vi "BRig_RT__Case_Exp__State_initTrial__LC_ENL__v3.vi"(6 "input_arrTrig":bool[](array[boolean]), 8 "input_dataTrial":u16[][](array[numeric]), 9 "input_dataExp":u16[](array[numeric]), 10 "input_dataLC":u16[](array[numeric]), 11 "input_dataCurrent":u16[](array[numeric])) -> (0 "output_dataTrial":u16[][](array[numeric]), 3 "output_dataCurrent":u16[](array[numeric]), 4 "output_arrTrig":bool[](array[boolean]))   [LabVIEW 2014]
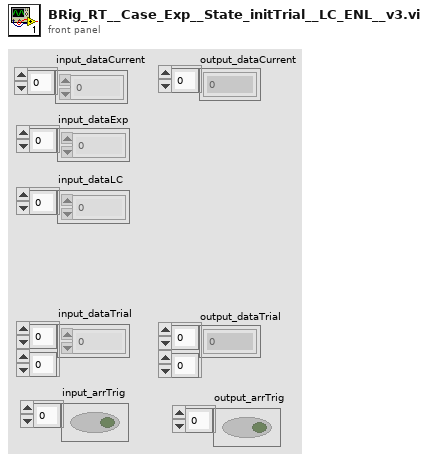
[diagram p1: front panel]
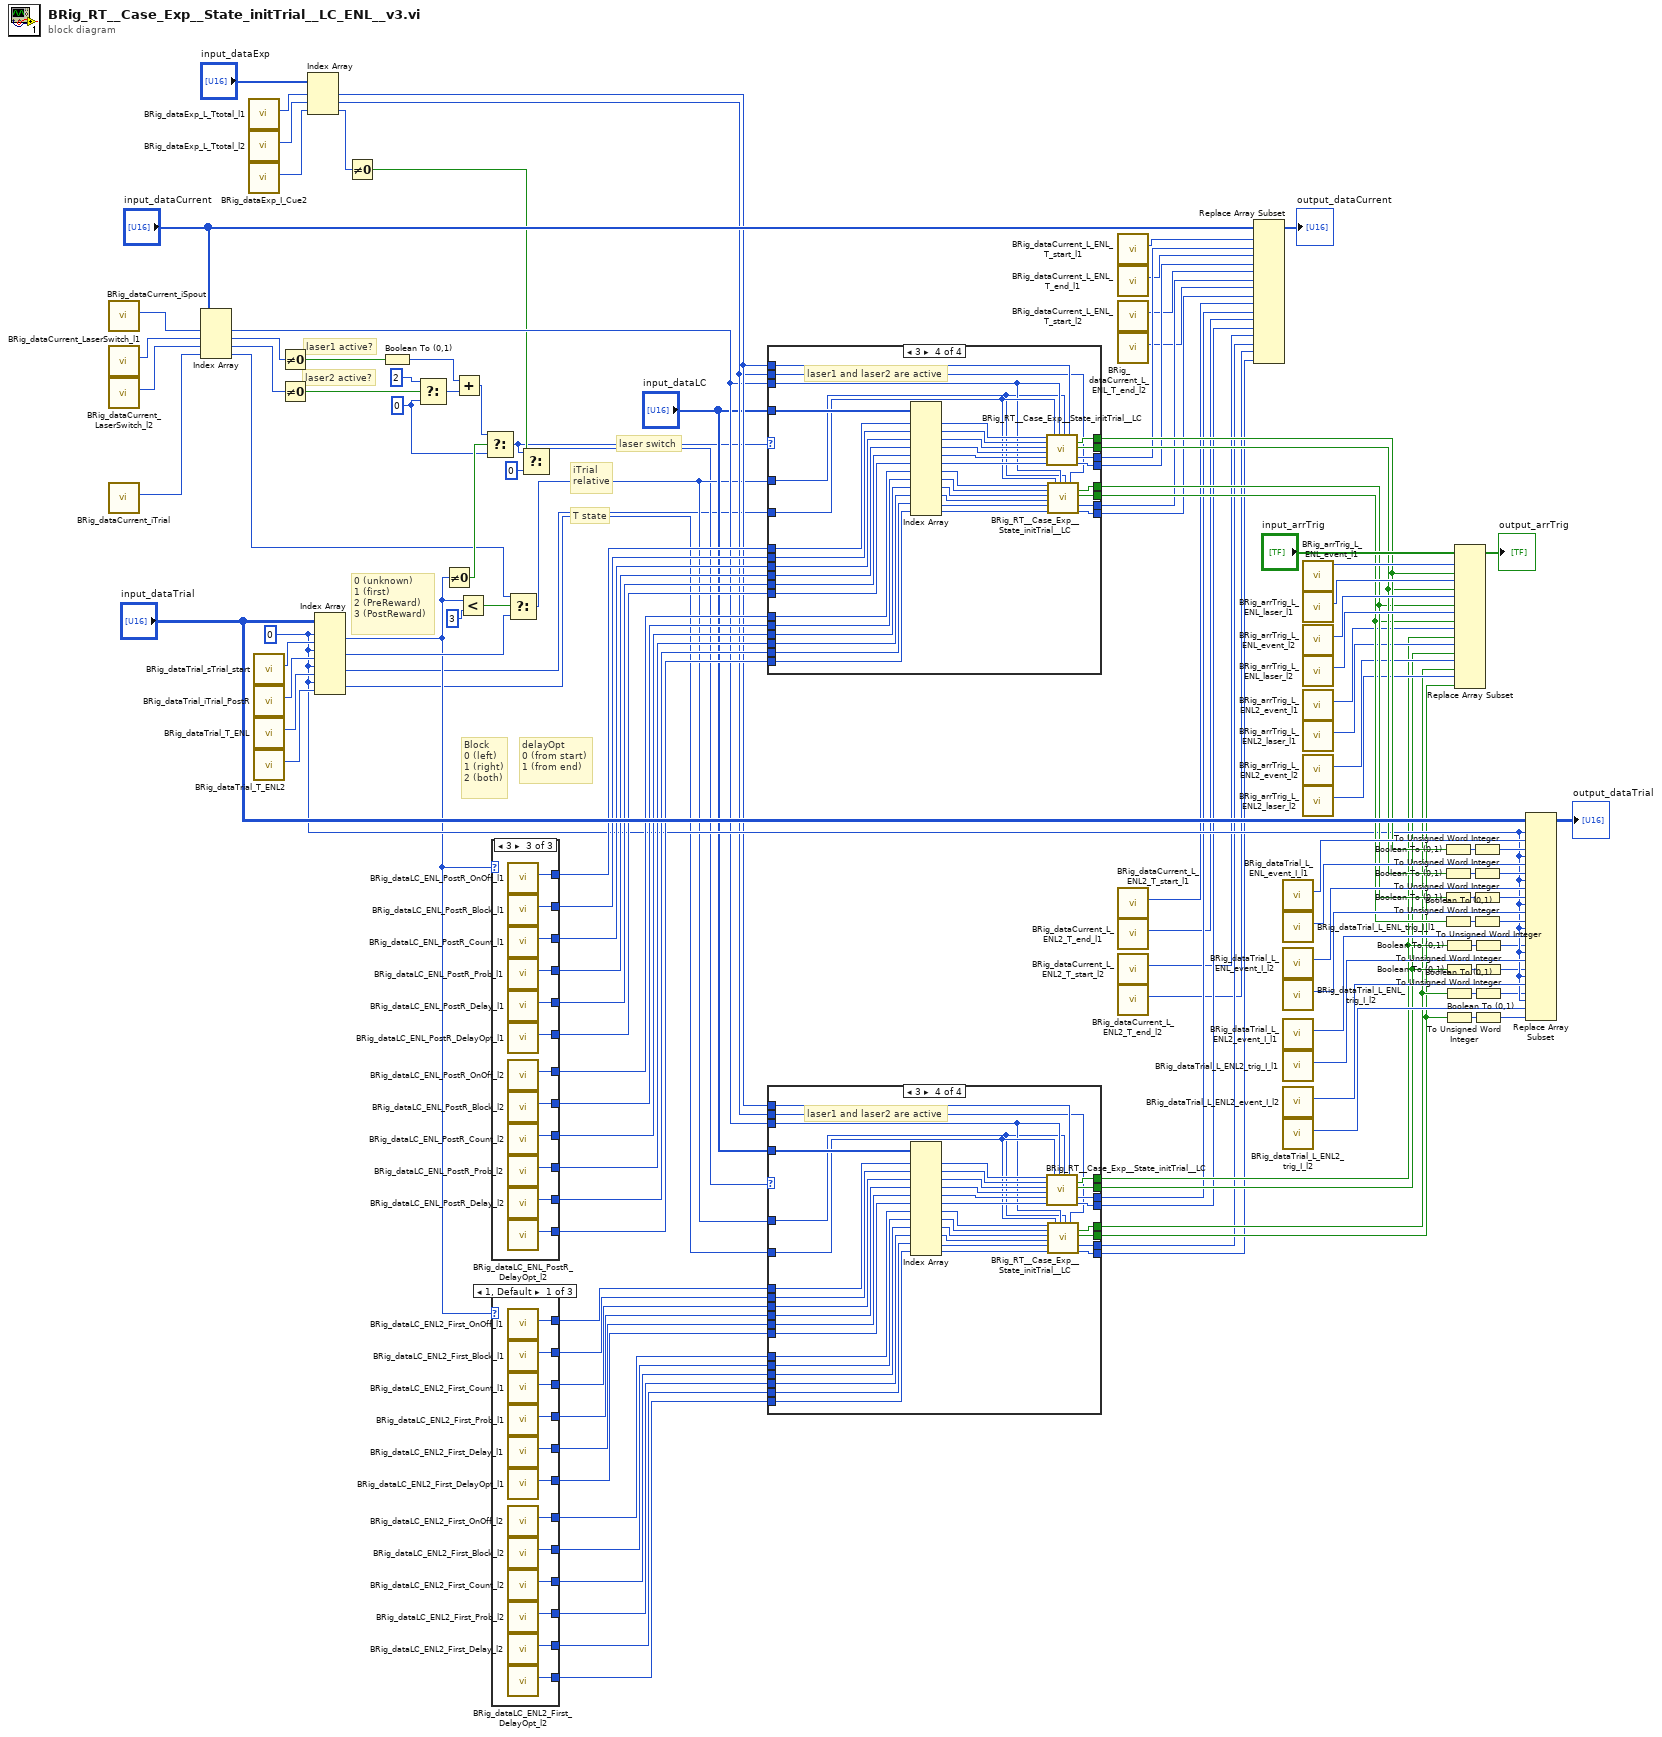
[diagram p0: block diagram]
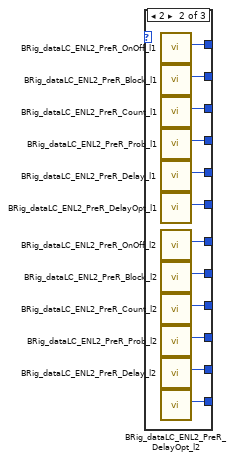
[diagram p2: hidden frame]
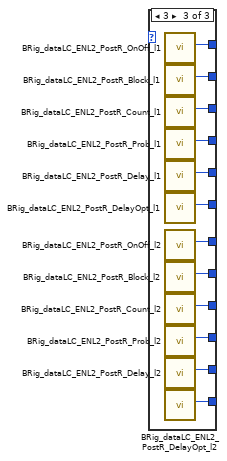
[diagram p3: hidden frame]
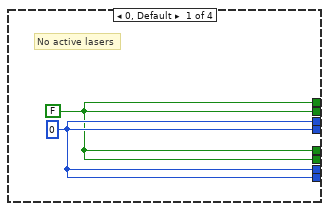
[diagram p4: hidden frame]
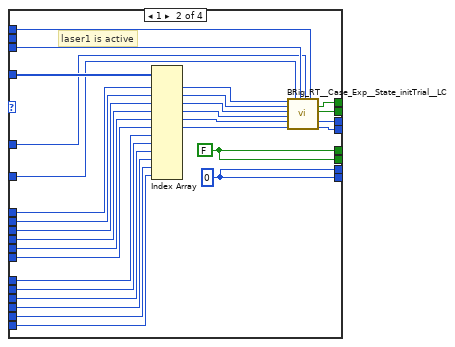
[diagram p5: hidden frame]
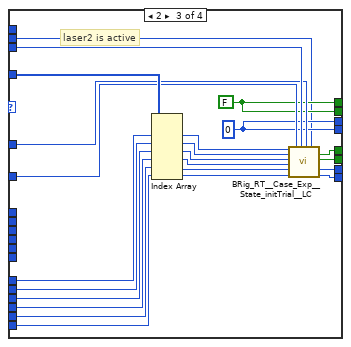
[diagram p6: hidden frame]
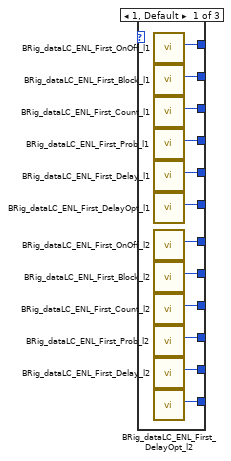
[diagram p7: hidden frame]
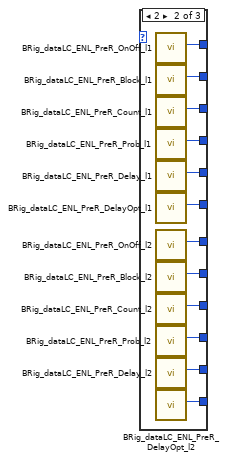
[diagram p8: hidden frame]
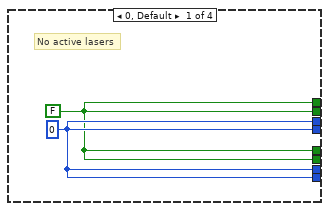
[diagram p9: hidden frame]
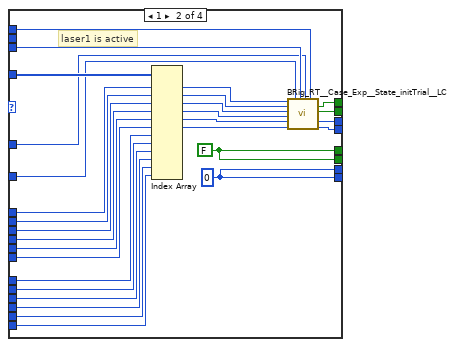
[diagram p10: hidden frame]
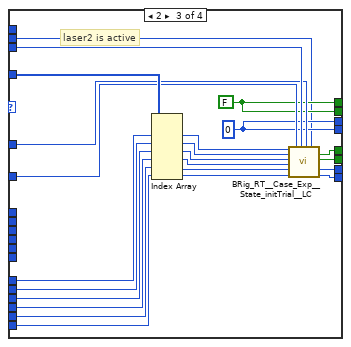
[diagram p11: hidden frame]
diagram:
  w44 = 0
  w115 = i16 0 ("f")
  # "iTrial\nrelative"
  # "laser switch"
  # "T state"
  # "delayOpt\n0 (from start)\n1 (from end)"
  # "Block\n0 (left)\n1 (right)\n2 (both)"
  # "0 (unknown)\n1 (first)\n2 (PreReward)\n3 (PostReward)"
  # "laser2 active?"
  # "laser1 active?"
  n1 = call "BRig_dataCurrent_iSpout.vi"() -> ("output_iSpout"=w113:i32)  [unwired: 11 in]
  n2 = call "BRig_dataCurrent_LaserSwitch_l1.vi"() -> ("output_LaserSwitch_l1"=w126:i32)  [unwired: 11 in]
  n3 = call "BRig_dataCurrent_LaserSwitch_l2.vi"() -> ("output_LaserSwitch_l2"=w125:i32)  [unwired: 11 in]
  n4 = call "BRig_dataCurrent_iTrial.vi"() -> ("output_iTrial"=w58:i32)  [unwired: 11 in]
  n5 = Index Array(array="input_dataCurrent", index #1=w113, index #2=w126, index #3=w125, index #4=w58) -> (element #1=w36:u16, element #2=w124:u16, element #3=w123:u16, element #4=w57:u16)
  n6 = call "BRig_dataExp_L_Ttotal_l1.vi"() -> ("output_L_Ttotal_l1"=w64:i32)  [unwired: 11 in]
  n7 = call "BRig_dataExp_L_Ttotal_l2.vi"() -> ("output_L_Ttotal_l2"=w65:i32)  [unwired: 11 in]
  n8 = call "BRig_dataExp_I_Cue2.vi"() -> ("output_I_Cue2"=w8:i32)  [unwired: 11 in]
  n9 = call "BRig_dataTrial_sTrial_start.vi"() -> ("output_sTrial_start"=w122:i32)  [unwired: 11 in]
  n10 = call "BRig_dataTrial_iTrial_PostR.vi"() -> ("output_iTrial_PostR"=w61:i32)  [unwired: 11 in]
  n11 = call "BRig_dataTrial_T_ENL.vi"() -> ("output_T_ENL"=w62:i32)  [unwired: 11 in]
  n12 = call "BRig_dataTrial_T_ENL2.vi"() -> ("output_T_ENL2"=w56:i32)  [unwired: 11 in]
  n13 = Not Equal To 0?(x=w124) -> (x != 0?=w121:bool)
  n14 = Not Equal To 0?(x=w123) -> (x != 0?=w120:bool)
  n15 = Index Array(array="input_dataExp", index #1=w64, index #2=w65, index #3=w8) -> (element #1=w38:u16, element #2=w37:u16, element #3=w7:u16)
  n16 = Index Array(array="input_dataTrial", index (row) #1=w44, index (col) #1=w122, index (row) #2=w44, index (col) #2=w61, index (row) #3=w44, index (col) #3=w62, index (row) #4=w44, index (col) #4=w56) -> (element #1=w33:u16, element #2=w59:u16, element #3=w2:u16, element #4=w1:u16)
  n17 = Not Equal To 0?(x=w7) -> (x != 0?=w6:bool)
  n18 = Boolean To (0,1)(Boolean=w121) -> (0, 1=w117:i16)
  n19 = Select(t=i16 2, s=w120, f=w115) -> (s? t:f=w118:i16)
  n20 = Not Equal To 0?(x=w33) -> (x != 0?=w116:bool)
  n21 = Add(x=w117, y=w118) -> (x+y=w114:i16)
  n22 = Less?(x=w33, y=u16 3) -> (x < y?=w60:bool)
  n23 = Select(t=w114, s=w116, f=w115) -> (s? t:f=w4:i16)
  n24 = case shown="3" w33 {
    tunnel: [w138 w150 w162] -> w77
    tunnel: [w137 w149 w151] -> w76
    tunnel: [w136 w148 w152] -> w75
    tunnel: [w135 w147 w153] -> w74
    tunnel: [w134 w146 w154] -> w73
    tunnel: [w133 w145 w155] -> w72
    tunnel: [w132 w144 w161] -> w71
    tunnel: [w131 w143 w160] -> w70
    tunnel: [w130 w142 w159] -> w69
    tunnel: [w129 w141 w158] -> w68
    tunnel: [w128 w140 w157] -> w67
    tunnel: [w127 w139 w156] -> w66
    frame 1, Default {
      n25 = call "BRig_dataLC_ENL_First_OnOff_l1.vi"() -> ("output_ENL_First_OnOff"=w138:i32)  [unwired: 11 in]
      n26 = call "BRig_dataLC_ENL_First_Block_l1.vi"() -> ("output_ENL_First_Block"=w137:i32)  [unwired: 11 in]
      n27 = call "BRig_dataLC_ENL_First_Count_l1.vi"() -> ("output_ENL_First_Count"=w136:i32)  [unwired: 11 in]
      n28 = call "BRig_dataLC_ENL_First_Prob_l1.vi"() -> ("output_ENL_First_Prob"=w135:i32)  [unwired: 11 in]
      n29 = call "BRig_dataLC_ENL_First_Delay_l1.vi"() -> ("output_ENL_First_Delay"=w134:i32)  [unwired: 11 in]
      n30 = call "BRig_dataLC_ENL_First_DelayOpt_l1.vi"() -> ("output_ENL_First_DelayOpt"=w133:i32)  [unwired: 11 in]
      n31 = call "BRig_dataLC_ENL_First_OnOff_l2.vi"() -> ("output_ENL_First_OnOff_l2"=w132:i32)  [unwired: 11 in]
      n32 = call "BRig_dataLC_ENL_First_Block_l2.vi"() -> ("output_ENL_First_Block_l2"=w131:i32)  [unwired: 11 in]
      n33 = call "BRig_dataLC_ENL_First_Count_l2.vi"() -> ("output_ENL_First_Count_l2"=w130:i32)  [unwired: 11 in]
      n34 = call "BRig_dataLC_ENL_First_Prob_l2.vi"() -> ("output_ENL_First_Prob_l2"=w129:i32)  [unwired: 11 in]
      n35 = call "BRig_dataLC_ENL_First_Delay_l2.vi"() -> ("output_ENL_First_Delay_l2"=w128:i32)  [unwired: 11 in]
      n36 = call "BRig_dataLC_ENL_First_DelayOpt_l2.vi"() -> ("output_ENL_First_DelayOpt_l2"=w127:i32)  [unwired: 11 in]
    }
    frame 2 {
      n37 = call "BRig_dataLC_ENL_PreR_OnOff_l1.vi"() -> ("output_ENL_PreR_OnOff"=w150:i32)  [unwired: 11 in]
      n38 = call "BRig_dataLC_ENL_PreR_Block_l1.vi"() -> ("output_ENL_PreR_Block"=w149:i32)  [unwired: 11 in]
      n39 = call "BRig_dataLC_ENL_PreR_Count_l1.vi"() -> ("output_ENL_PreR_Count"=w148:i32)  [unwired: 11 in]
      n40 = call "BRig_dataLC_ENL_PreR_Prob_l1.vi"() -> ("output_ENL_PreR_Prob"=w147:i32)  [unwired: 11 in]
      n41 = call "BRig_dataLC_ENL_PreR_Delay_l1.vi"() -> ("output_ENL_PreR_Delay"=w146:i32)  [unwired: 11 in]
      n42 = call "BRig_dataLC_ENL_PreR_DelayOpt_l1.vi"() -> ("output_ENL_PreR_DelayOpt"=w145:i32)  [unwired: 11 in]
      n43 = call "BRig_dataLC_ENL_PreR_OnOff_l2.vi"() -> ("output_ENL_PreR_OnOff_l2"=w144:i32)  [unwired: 11 in]
      n44 = call "BRig_dataLC_ENL_PreR_Block_l2.vi"() -> ("output_ENL_PreR_Block_l2"=w143:i32)  [unwired: 11 in]
      n45 = call "BRig_dataLC_ENL_PreR_Count_l2.vi"() -> ("output_ENL_PreR_Count_l2"=w142:i32)  [unwired: 11 in]
      n46 = call "BRig_dataLC_ENL_PreR_Prob_l2.vi"() -> ("output_ENL_PreR_Prob_l2"=w141:i32)  [unwired: 11 in]
      n47 = call "BRig_dataLC_ENL_PreR_Delay_l2.vi"() -> ("output_ENL_PreR_Delay_l2"=w140:i32)  [unwired: 11 in]
      n48 = call "BRig_dataLC_ENL_PreR_DelayOpt_l2.vi"() -> ("output_ENL_PreR_DelayOpt_l2"=w139:i32)  [unwired: 11 in]
    }
    frame 3 {
      n49 = call "BRig_dataLC_ENL_PostR_OnOff_l1.vi"() -> ("output_ENL_PostR_OnOff"=w162:i32)  [unwired: 11 in]
      n50 = call "BRig_dataLC_ENL_PostR_Block_l1.vi"() -> ("output_ENL_PostR_Block"=w151:i32)  [unwired: 11 in]
      n51 = call "BRig_dataLC_ENL_PostR_Count_l1.vi"() -> ("output_ENL_PostR_Count"=w152:i32)  [unwired: 11 in]
      n52 = call "BRig_dataLC_ENL_PostR_Prob_l1.vi"() -> ("output_ENL_PostR_Prob"=w153:i32)  [unwired: 11 in]
      n53 = call "BRig_dataLC_ENL_PostR_Delay_l1.vi"() -> ("output_ENL_PostR_Delay"=w154:i32)  [unwired: 11 in]
      n54 = call "BRig_dataLC_ENL_PostR_DelayOpt_l1.vi"() -> ("output_ENL_PostR_DelayOpt"=w155:i32)  [unwired: 11 in]
      n55 = call "BRig_dataLC_ENL_PostR_OnOff_l2.vi"() -> ("output_ENL_PostR_OnOff_l2"=w161:i32)  [unwired: 11 in]
      n56 = call "BRig_dataLC_ENL_PostR_Block_l2.vi"() -> ("output_ENL_PostR_Block_l2"=w160:i32)  [unwired: 11 in]
      n57 = call "BRig_dataLC_ENL_PostR_Count_l2.vi"() -> ("output_ENL_PostR_Count_l2"=w159:i32)  [unwired: 11 in]
      n58 = call "BRig_dataLC_ENL_PostR_Prob_l2.vi"() -> ("output_ENL_PostR_Prob_l2"=w158:i32)  [unwired: 11 in]
      n59 = call "BRig_dataLC_ENL_PostR_Delay_l2.vi"() -> ("output_ENL_PostR_Delay_l2"=w157:i32)  [unwired: 11 in]
      n60 = call "BRig_dataLC_ENL_PostR_DelayOpt_l2.vi"() -> ("output_ENL_PostR_DelayOpt_l2"=w156:i32)  [unwired: 11 in]
    }
  }
  n61 = case shown="1, Default" w33 {
    tunnel: [w174 w186 w198] -> w32
    tunnel: [w173 w185 w197] -> w31
    tunnel: [w172 w184 w196] -> w30
    tunnel: [w171 w183 w195] -> w29
    tunnel: [w170 w182 w194] -> w28
    tunnel: [w169 w181 w193] -> w27
    tunnel: [w168 w180 w192] -> w26
    tunnel: [w167 w179 w191] -> w25
    tunnel: [w166 w178 w190] -> w24
    tunnel: [w165 w177 w189] -> w23
    tunnel: [w164 w176 w188] -> w22
    tunnel: [w163 w175 w187] -> w21
    frame 1, Default {
      n62 = call "BRig_dataLC_ENL2_First_OnOff_l1.vi"() -> ("output_ENL2_First_OnOff"=w174:i32)  [unwired: 11 in]
      n63 = call "BRig_dataLC_ENL2_First_Block_l1.vi"() -> ("output_ENL2_First_Block"=w173:i32)  [unwired: 11 in]
      n64 = call "BRig_dataLC_ENL2_First_Count_l1.vi"() -> ("output_ENL2_First_Count"=w172:i32)  [unwired: 11 in]
      n65 = call "BRig_dataLC_ENL2_First_Prob_l1.vi"() -> ("output_ENL2_First_Prob"=w171:i32)  [unwired: 11 in]
      n66 = call "BRig_dataLC_ENL2_First_Delay_l1.vi"() -> ("output_ENL2_First_Delay"=w170:i32)  [unwired: 11 in]
      n67 = call "BRig_dataLC_ENL2_First_DelayOpt_l1.vi"() -> ("output_ENL2_First_DelayOpt"=w169:i32)  [unwired: 11 in]
      n68 = call "BRig_dataLC_ENL2_First_OnOff_l2.vi"() -> ("output_ENL2_First_OnOff_l2"=w168:i32)  [unwired: 11 in]
      n69 = call "BRig_dataLC_ENL2_First_Block_l2.vi"() -> ("output_ENL2_First_Block_l2"=w167:i32)  [unwired: 11 in]
      n70 = call "BRig_dataLC_ENL2_First_Count_l2.vi"() -> ("output_ENL2_First_Count_l2"=w166:i32)  [unwired: 11 in]
      n71 = call "BRig_dataLC_ENL2_First_Prob_l2.vi"() -> ("output_ENL2_First_Prob_l2"=w165:i32)  [unwired: 11 in]
      n72 = call "BRig_dataLC_ENL2_First_Delay_l2.vi"() -> ("output_ENL2_First_Delay_l2"=w164:i32)  [unwired: 11 in]
      n73 = call "BRig_dataLC_ENL2_First_DelayOpt_l2.vi"() -> ("output_ENL2_First_DelayOpt_l2"=w163:i32)  [unwired: 11 in]
    }
    frame 2 {
      n74 = call "BRig_dataLC_ENL2_PreR_OnOff_l1.vi"() -> ("output_ENL2_PreR_OnOff"=w186:i32)  [unwired: 11 in]
      n75 = call "BRig_dataLC_ENL2_PreR_Block_l1.vi"() -> ("output_ENL2_PreR_Block"=w185:i32)  [unwired: 11 in]
      n76 = call "BRig_dataLC_ENL2_PreR_Count_l1.vi"() -> ("output_ENL2_PreR_Count"=w184:i32)  [unwired: 11 in]
      n77 = call "BRig_dataLC_ENL2_PreR_Prob_l1.vi"() -> ("output_ENL2_PreR_Prob"=w183:i32)  [unwired: 11 in]
      n78 = call "BRig_dataLC_ENL2_PreR_Delay_l1.vi"() -> ("output_ENL2_PreR_Delay"=w182:i32)  [unwired: 11 in]
      n79 = call "BRig_dataLC_ENL2_PreR_DelayOpt_l1.vi"() -> ("output_ENL2_PreR_DelayOpt"=w181:i32)  [unwired: 11 in]
      n80 = call "BRig_dataLC_ENL2_PreR_OnOff_l2.vi"() -> ("output_ENL2_PreR_OnOff_l2"=w180:i32)  [unwired: 11 in]
      n81 = call "BRig_dataLC_ENL2_PreR_Block_l2.vi"() -> ("output_ENL2_PreR_Block_l2"=w179:i32)  [unwired: 11 in]
      n82 = call "BRig_dataLC_ENL2_PreR_Count_l2.vi"() -> ("output_ENL2_PreR_Count_l2"=w178:i32)  [unwired: 11 in]
      n83 = call "BRig_dataLC_ENL2_PreR_Prob_l2.vi"() -> ("output_ENL2_PreR_Prob_l2"=w177:i32)  [unwired: 11 in]
      n84 = call "BRig_dataLC_ENL2_PreR_Delay_l2.vi"() -> ("output_ENL2_PreR_Delay_l2"=w176:i32)  [unwired: 11 in]
      n85 = call "BRig_dataLC_ENL2_PreR_DelayOpt_l2.vi"() -> ("output_ENL2_PreR_DelayOpt_l2"=w175:i32)  [unwired: 11 in]
    }
    frame 3 {
      n86 = call "BRig_dataLC_ENL2_PostR_OnOff_l1.vi"() -> ("output_ENL2_PostR_OnOff"=w198:i32)  [unwired: 11 in]
      n87 = call "BRig_dataLC_ENL2_PostR_Block_l1.vi"() -> ("output_ENL2_PostR_Block"=w197:i32)  [unwired: 11 in]
      n88 = call "BRig_dataLC_ENL2_PostR_Count_l1.vi"() -> ("output_ENL2_PostR_Count"=w196:i32)  [unwired: 11 in]
      n89 = call "BRig_dataLC_ENL2_PostR_Prob_l1.vi"() -> ("output_ENL2_PostR_Prob"=w195:i32)  [unwired: 11 in]
      n90 = call "BRig_dataLC_ENL2_PostR_Delay_l1.vi"() -> ("output_ENL2_PostR_Delay"=w194:i32)  [unwired: 11 in]
      n91 = call "BRig_dataLC_ENL2_PostR_DelayOpt_l1.vi"() -> ("output_ENL2_PostR_DelayOpt"=w193:i32)  [unwired: 11 in]
      n92 = call "BRig_dataLC_ENL2_PostR_OnOff_l2.vi"() -> ("output_ENL2_PostR_OnOff_l2"=w192:i32)  [unwired: 11 in]
      n93 = call "BRig_dataLC_ENL2_PostR_Block_l2.vi"() -> ("output_ENL2_PostR_Block_l2"=w191:i32)  [unwired: 11 in]
      n94 = call "BRig_dataLC_ENL2_PostR_Count_l2.vi"() -> ("output_ENL2_PostR_Count_l2"=w190:i32)  [unwired: 11 in]
      n95 = call "BRig_dataLC_ENL2_PostR_Prob_l2.vi"() -> ("output_ENL2_PostR_Prob_l2"=w189:i32)  [unwired: 11 in]
      n96 = call "BRig_dataLC_ENL2_PostR_Delay_l2.vi"() -> ("output_ENL2_PostR_Delay_l2"=w188:i32)  [unwired: 11 in]
      n97 = call "BRig_dataLC_ENL2_PostR_DelayOpt_l2.vi"() -> ("output_ENL2_PostR_DelayOpt_l2"=w187:i32)  [unwired: 11 in]
    }
  }
  n98 = Select(t=w57, s=w60, f=w59) -> (s? t:f=w34:u16)
  n99 = Select(t=w4, s=w6, f=i16 0) -> (s? t:f=w3:i16)
  n100 = case shown="3" w4 {
    tunnel: "input_dataLC" -> [_ w229 w252 w290]
    tunnel: w36 -> [_ w221 w244 w276]
    tunnel: w2 -> [_ w222 w245 w277]
    tunnel: w34 -> [_ w220 w243 w275]
    tunnel: [w199 w219 w232 w274] -> w99
    tunnel: [w199 w218 w232 w273] -> w93
    tunnel: [w200 w217 w231 w272] -> w84
    tunnel: [w200 w216 w231 w271] -> w82
    tunnel: [w199 w203 w242 w270] -> w89
    tunnel: [w200 w202 w241 w269] -> w80
    tunnel: [w199 w203 w240 w268] -> w91
    tunnel: [w200 w202 w239 w267] -> w78
    tunnel: w77 -> [_ w215 _ w266]
    tunnel: w76 -> [_ w214 _ w265]
    tunnel: w75 -> [_ w213 _ w264]
    tunnel: w74 -> [_ w212 _ w263]
    tunnel: w73 -> [_ w211 _ w262]
    tunnel: w72 -> [_ w210 _ w261]
    tunnel: w71 -> [_ w209 w238 w260]
    tunnel: w70 -> [_ w208 w237 w259]
    tunnel: w69 -> [_ w207 w236 w258]
    tunnel: w68 -> [_ w206 w235 w257]
    tunnel: w67 -> [_ w205 w234 w256]
    tunnel: w66 -> [_ w204 w233 w255]
    tunnel: w38 -> [_ w201 _ w254]
    tunnel: w37 -> [_ _ w230 w253]
    frame 0, Default {
      w200 = u16 0
      w199 = FALSE
      # "No active lasers"
    }
    frame 1 {
      w202 = u16 0
      w203 = FALSE
      # "laser1 is active"
      n101 = Index Array(array=w229, index #1=w215, index #2=w214, index #3=w213, index #4=w212, index #5=w211, index #6=w210, index #7=w209, index #8=w208, index #9=w207, index #10=w206, index #11=w205, index #12=w204) -> (element #1=w228:u16, element #2=w227:u16, element #3=w226:u16, element #4=w225:u16, element #5=w224:u16, element #6=w223:u16)  [unwired: 6 out]
      n102 = call "BRig_RT__Case_Exp__State_initTrial__LC.vi"("input_L_OnOff"=w228, "input_L_Block"=w227, "input_L_Count"=w226, "input_L_Prob"=w225, "input_L_Tdelay"=w224, "input_L_delayOpt"=w223, "input_T_state"=w222, "input_iSpout"=w221, "input_iTrial_relative"=w220, "input_L_T"=w201) -> ("output_LC_Event"=w219:bool, "output_LC_Laser"=w218:bool, "output_L_Tstart"=w217:u16, "output_L_Tend"=w216:u16)  [unwired: 6 in]
    }
    frame 2 {
      w231 = u16 0
      w232 = FALSE
      # "laser2 is active"
      n103 = Index Array(array=w252, index #1=w238, index #2=w237, index #3=w236, index #4=w235, index #5=w234, index #6=w233) -> (element #1=w246:u16, element #2=w247:u16, element #3=w248:u16, element #4=w249:u16, element #5=w250:u16, element #6=w251:u16)
      n104 = call "BRig_RT__Case_Exp__State_initTrial__LC.vi"("input_L_OnOff"=w246, "input_L_Block"=w247, "input_L_Count"=w248, "input_L_Prob"=w249, "input_L_Tdelay"=w250, "input_L_delayOpt"=w251, "input_T_state"=w245, "input_iSpout"=w244, "input_iTrial_relative"=w243, "input_L_T"=w230) -> ("output_LC_Event"=w240:bool, "output_LC_Laser"=w242:bool, "output_L_Tstart"=w241:u16, "output_L_Tend"=w239:u16)  [unwired: 6 in]
    }
    frame 3 {
      # "laser1 and laser2 are active"
      n105 = Index Array(array=w290, index #1=w266, index #2=w265, index #3=w264, index #4=w263, index #5=w262, index #6=w261, index #7=w260, index #8=w259, index #9=w258, index #10=w257, index #11=w256, index #12=w255) -> (element #1=w289:u16, element #2=w288:u16, element #3=w287:u16, element #4=w286:u16, element #5=w285:u16, element #6=w284:u16, element #7=w278:u16, element #8=w279:u16, element #9=w280:u16, element #10=w281:u16, element #11=w282:u16, element #12=w283:u16)
      n106 = call "BRig_RT__Case_Exp__State_initTrial__LC.vi"("input_L_OnOff"=w289, "input_L_Block"=w288, "input_L_Count"=w287, "input_L_Prob"=w286, "input_L_Tdelay"=w285, "input_L_delayOpt"=w284, "input_T_state"=w277, "input_iSpout"=w276, "input_iTrial_relative"=w275, "input_L_T"=w254) -> ("output_LC_Event"=w274:bool, "output_LC_Laser"=w273:bool, "output_L_Tstart"=w272:u16, "output_L_Tend"=w271:u16)  [unwired: 6 in]
      n107 = call "BRig_RT__Case_Exp__State_initTrial__LC.vi"("input_L_OnOff"=w278, "input_L_Block"=w279, "input_L_Count"=w280, "input_L_Prob"=w281, "input_L_Tdelay"=w282, "input_L_delayOpt"=w283, "input_T_state"=w277, "input_iSpout"=w276, "input_iTrial_relative"=w275, "input_L_T"=w253) -> ("output_LC_Event"=w268:bool, "output_LC_Laser"=w270:bool, "output_L_Tstart"=w269:u16, "output_L_Tend"=w267:u16)  [unwired: 6 in]
    }
  }
  n108 = case shown="3" w3 {
    tunnel: "input_dataLC" -> [_ w321 w344 w382]
    tunnel: w36 -> [_ w313 w336 w368]
    tunnel: w1 -> [_ w314 w337 w369]
    tunnel: w34 -> [_ w312 w335 w367]
    tunnel: [w291 w311 w324 w366] -> w20
    tunnel: [w291 w310 w324 w365] -> w19
    tunnel: [w292 w309 w323 w364] -> w15
    tunnel: [w292 w308 w323 w363] -> w13
    tunnel: [w291 w295 w334 w362] -> w17
    tunnel: [w292 w294 w333 w361] -> w11
    tunnel: [w291 w295 w332 w360] -> w18
    tunnel: [w292 w294 w331 w359] -> w9
    tunnel: w32 -> [_ w307 _ w358]
    tunnel: w31 -> [_ w306 _ w357]
    tunnel: w30 -> [_ w305 _ w356]
    tunnel: w29 -> [_ w304 _ w355]
    tunnel: w28 -> [_ w303 _ w354]
    tunnel: w27 -> [_ w302 _ w353]
    tunnel: w26 -> [_ w301 w330 w352]
    tunnel: w25 -> [_ w300 w329 w351]
    tunnel: w24 -> [_ w299 w328 w350]
    tunnel: w23 -> [_ w298 w327 w349]
    tunnel: w22 -> [_ w297 w326 w348]
    tunnel: w21 -> [_ w296 w325 w347]
    tunnel: w38 -> [_ w293 _ w346]
    tunnel: w37 -> [_ _ w322 w345]
    frame 0, Default {
      w292 = u16 0
      w291 = FALSE
      # "No active lasers"
    }
    frame 1 {
      w294 = u16 0
      w295 = FALSE
      # "laser1 is active"
      n109 = Index Array(array=w321, index #1=w307, index #2=w306, index #3=w305, index #4=w304, index #5=w303, index #6=w302, index #7=w301, index #8=w300, index #9=w299, index #10=w298, index #11=w297, index #12=w296) -> (element #1=w320:u16, element #2=w319:u16, element #3=w318:u16, element #4=w317:u16, element #5=w316:u16, element #6=w315:u16)  [unwired: 6 out]
      n110 = call "BRig_RT__Case_Exp__State_initTrial__LC.vi"("input_L_OnOff"=w320, "input_L_Block"=w319, "input_L_Count"=w318, "input_L_Prob"=w317, "input_L_Tdelay"=w316, "input_L_delayOpt"=w315, "input_T_state"=w314, "input_iSpout"=w313, "input_iTrial_relative"=w312, "input_L_T"=w293) -> ("output_LC_Event"=w311:bool, "output_LC_Laser"=w310:bool, "output_L_Tstart"=w309:u16, "output_L_Tend"=w308:u16)  [unwired: 6 in]
    }
    frame 2 {
      w323 = u16 0
      w324 = FALSE
      # "laser2 is active"
      n111 = Index Array(array=w344, index #1=w330, index #2=w329, index #3=w328, index #4=w327, index #5=w326, index #6=w325) -> (element #1=w338:u16, element #2=w339:u16, element #3=w340:u16, element #4=w341:u16, element #5=w342:u16, element #6=w343:u16)
      n112 = call "BRig_RT__Case_Exp__State_initTrial__LC.vi"("input_L_OnOff"=w338, "input_L_Block"=w339, "input_L_Count"=w340, "input_L_Prob"=w341, "input_L_Tdelay"=w342, "input_L_delayOpt"=w343, "input_T_state"=w337, "input_iSpout"=w336, "input_iTrial_relative"=w335, "input_L_T"=w322) -> ("output_LC_Event"=w332:bool, "output_LC_Laser"=w334:bool, "output_L_Tstart"=w333:u16, "output_L_Tend"=w331:u16)  [unwired: 6 in]
    }
    frame 3 {
      # "laser1 and laser2 are active"
      n113 = Index Array(array=w382, index #1=w358, index #2=w357, index #3=w356, index #4=w355, index #5=w354, index #6=w353, index #7=w352, index #8=w351, index #9=w350, index #10=w349, index #11=w348, index #12=w347) -> (element #1=w381:u16, element #2=w380:u16, element #3=w379:u16, element #4=w378:u16, element #5=w377:u16, element #6=w376:u16, element #7=w370:u16, element #8=w371:u16, element #9=w372:u16, element #10=w373:u16, element #11=w374:u16, element #12=w375:u16)
      n114 = call "BRig_RT__Case_Exp__State_initTrial__LC.vi"("input_L_OnOff"=w381, "input_L_Block"=w380, "input_L_Count"=w379, "input_L_Prob"=w378, "input_L_Tdelay"=w377, "input_L_delayOpt"=w376, "input_T_state"=w369, "input_iSpout"=w368, "input_iTrial_relative"=w367, "input_L_T"=w346) -> ("output_LC_Event"=w366:bool, "output_LC_Laser"=w365:bool, "output_L_Tstart"=w364:u16, "output_L_Tend"=w363:u16)  [unwired: 6 in]
      n115 = call "BRig_RT__Case_Exp__State_initTrial__LC.vi"("input_L_OnOff"=w370, "input_L_Block"=w371, "input_L_Count"=w372, "input_L_Prob"=w373, "input_L_Tdelay"=w374, "input_L_delayOpt"=w375, "input_T_state"=w369, "input_iSpout"=w368, "input_iTrial_relative"=w367, "input_L_T"=w345) -> ("output_LC_Event"=w360:bool, "output_LC_Laser"=w362:bool, "output_L_Tstart"=w361:u16, "output_L_Tend"=w359:u16)  [unwired: 6 in]
    }
  }
  n116 = call "BRig_dataCurrent_L_ENL_T_start_l1.vi"() -> ("output_L_ENL_T_start_l1"=w85:i32)  [unwired: 11 in]
  n117 = call "BRig_dataCurrent_L_ENL_T_end_l1.vi"() -> ("output_L_ENL_T_end_l1"=w83:i32)  [unwired: 11 in]
  n118 = call "BRig_dataCurrent_L_ENL_T_start_l2.vi"() -> ("output_L_T_ENL1_start_l2"=w81:i32)  [unwired: 11 in]
  n119 = call "BRig_dataCurrent_L_ENL_T_end_l2.vi"() -> ("output_L_ENL_T_end_l2"=w79:i32)  [unwired: 11 in]
  n120 = call "BRig_dataCurrent_L_ENL2_T_start_l1.vi"() -> ("output_L_ENL2_T_start_l1"=w16:i32)  [unwired: 11 in]
  n121 = call "BRig_dataCurrent_L_ENL2_T_end_l1.vi"() -> ("output_L_ENL2_T_end_l1"=w14:i32)  [unwired: 11 in]
  n122 = call "BRig_dataCurrent_L_ENL2_T_start_l2.vi"() -> ("output_L_T_ENL2_start_l2"=w12:i32)  [unwired: 11 in]
  n123 = call "BRig_dataCurrent_L_ENL2_T_end_l2.vi"() -> ("output_L_ENL2_T_end_l2"=w10:i32)  [unwired: 11 in]
  n124 = Replace Array Subset(array="input_dataCurrent", new element #1=w84, index #1=w85, new element #2=w82, index #2=w83, new element #3=w80, index #3=w81, new element #4=w78, index #4=w79, new element #5=w15, index #5=w16, new element #6=w13, index #6=w14, new element #7=w11, index #7=w12, new element #8=w9, index #8=w10) -> (→"output_dataCurrent":u16[])
  n125 = call "BRig_dataTrial_L_ENL_event_I_l1.vi"() -> ("output_L_ENL_event_I_l1"=w100:i32)  [unwired: 11 in]
  n126 = call "BRig_dataTrial_L_ENL_trig_I_l1.vi"() -> ("output_L_ENL_trig_I_l1"=w97:i32)  [unwired: 11 in]
  n127 = call "BRig_dataTrial_L_ENL_event_I_l2.vi"() -> ("output_L_ENL_event_I_l2"=w96:i32)  [unwired: 11 in]
  n128 = call "BRig_dataTrial_L_ENL_trig_I_l2.vi"() -> ("output_L_ENL_trig_I_l2"=w95:i32)  [unwired: 11 in]
  n129 = call "BRig_dataTrial_L_ENL2_event_I_l1.vi"() -> ("output_L_ENL2_event_I_l1"=w47:i32)  [unwired: 11 in]
  n130 = call "BRig_dataTrial_L_ENL2_trig_I_l1.vi"() -> ("output_L_ENL2_trig_I_l1"=w46:i32)  [unwired: 11 in]
  n131 = call "BRig_dataTrial_L_ENL2_event_I_l2.vi"() -> ("output_L_ENL2_event_I_l2"=w45:i32)  [unwired: 11 in]
  n132 = call "BRig_dataTrial_L_ENL2_trig_I_l2.vi"() -> ("output_L_ENL2_trig_I_l2"=w43:i32)  [unwired: 11 in]
  n133 = call "BRig_arrTrig_L_ENL_event_l1.vi"() -> ("output_L_ENL_event_l1"=w109:i32)  [unwired: 11 in]
  n134 = call "BRig_arrTrig_L_ENL_laser_l1.vi"() -> ("output_L_ENL_laserTrig_l1"=w108:i32)  [unwired: 11 in]
  n135 = call "BRig_arrTrig_L_ENL_event_l2.vi"() -> ("output_L_ENL_event_l2"=w107:i32)  [unwired: 11 in]
  n136 = call "BRig_arrTrig_L_ENL_laser_l2.vi"() -> ("output_L_ENL_laserTrig_l2"=w106:i32)  [unwired: 11 in]
  n137 = call "BRig_arrTrig_L_ENL2_event_l1.vi"() -> ("output_L_ENL2_event_l1"=w55:i32)  [unwired: 11 in]
  n138 = call "BRig_arrTrig_L_ENL2_laser_l1.vi"() -> ("output_L_ENL2_laserTrig_l1"=w54:i32)  [unwired: 11 in]
  n139 = call "BRig_arrTrig_L_ENL2_event_l2.vi"() -> ("output_L_ENL2_event_l2"=w53:i32)  [unwired: 11 in]
  n140 = call "BRig_arrTrig_L_ENL2_laser_l2.vi"() -> ("output_L_ENL2_laserTrig_l2"=w52:i32)  [unwired: 11 in]
  n141 = Boolean To (0,1)(Boolean=w99) -> (0, 1=w105:i16)
  n142 = Boolean To (0,1)(Boolean=w93) -> (0, 1=w104:i16)
  n143 = Boolean To (0,1)(Boolean=w91) -> (0, 1=w102:i16)
  n144 = Boolean To (0,1)(Boolean=w89) -> (0, 1=w103:i16)
  n145 = Boolean To (0,1)(Boolean=w20) -> (0, 1=w51:i16)
  n146 = Boolean To (0,1)(Boolean=w19) -> (0, 1=w50:i16)
  n147 = Boolean To (0,1)(Boolean=w18) -> (0, 1=w48:i16)
  n148 = Boolean To (0,1)(Boolean=w17) -> (0, 1=w49:i16)
  n149 = Replace Array Subset(array="input_arrTrig", new element #1=w99, index #1=w109, new element #2=w93, index #2=w108, new element #3=w91, index #3=w107, new element #4=w89, index #4=w106, new element #5=w20, index #5=w55, new element #6=w19, index #6=w54, new element #7=w18, index #7=w53, new element #8=w17, index #8=w52) -> (→"output_arrTrig":bool[])
  n150 = To Unsigned Word Integer(number=w105) -> (unsigned 16bit integer=w98:u16)
  n151 = To Unsigned Word Integer(number=w104) -> (unsigned 16bit integer=w94:u16)
  n152 = To Unsigned Word Integer(number=w102) -> (unsigned 16bit integer=w92:u16)
  n153 = To Unsigned Word Integer(number=w103) -> (unsigned 16bit integer=w90:u16)
  n154 = To Unsigned Word Integer(number=w51) -> (unsigned 16bit integer=w42:u16)
  n155 = To Unsigned Word Integer(number=w50) -> (unsigned 16bit integer=w41:u16)
  n156 = To Unsigned Word Integer(number=w48) -> (unsigned 16bit integer=w40:u16)
  n157 = To Unsigned Word Integer(number=w49) -> (unsigned 16bit integer=w39:u16)
  n158 = Replace Array Subset(array="input_dataTrial", new element #1=w98, index (row) #1=w44, index (col) #1=w100, new element #2=w94, index (row) #2=w44, index (col) #2=w97, new element #3=w92, index (row) #3=w44, index (col) #3=w96, new element #4=w90, index (row) #4=w44, index (col) #4=w95, new element #5=w42, index (row) #5=w44, index (col) #5=w47, new element #6=w41, index (row) #6=w44, index (col) #6=w46, new element #7=w40, index (row) #7=w44, index (col) #7=w45, new element #8=w39, index (row) #8=w44, index (col) #8=w43) -> (→"output_dataTrial":u16[][])
